vi "new square 1.vi"(11 "Error In":errorcluster) -> ()   [LabVIEW 2019]
uses:
  <vilib>/Platform/TimedLoop/XDataNode/timing_clust.ctl
  <vilib>/Platform/TimedLoop/XDataNode/nitl_modes.ctl
  <vilib>/Platform/TimedLoop/XDataNode/wakeup.ctl
  Global.vi
  <vilib>/platform/TimedLoop/XDataNode/XDataNode.xnode
  <vilib>/Platform/TimedLoop/XDataNode/XDNodeRunTimeDep.lvlib
panel:
  out "x >= y?":bool
  in  "msec Delay":u32=500
  out "msec Low":dbl=400.0
  out "msec High":dbl=600.0
  out "Duty Cycle":dbl
  out "Frequency":dbl
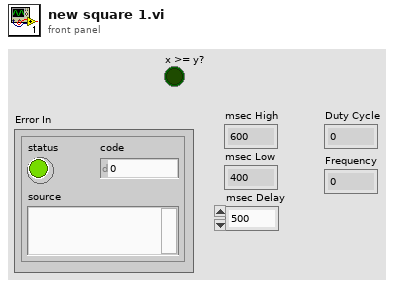
[diagram p1: front panel]
types:
  T1 = typedef "XDNodeRunTimeDep.lvlib/timing_clust.ctl" = cluster{"Expected End [f-1]":u64, "Actual End [f-1]":u64, "Finished Late? [f-1]":bool, "Expected End [i-1]":u64, "Actual End [i-1]":u64, "Finished Late? [i-1]":bool, "Expected Start [i]":u64, "Actual Start [i]":u64, "Expected Start [f]":u64, "Actual Start [f]":u64, "Source Name":string, "Structure Name":string, "Period":i64, "Deadline":i64, "Offset":i64, "Start":i64, "Priority":i32, "Timeout":i32, "Mode":T2, "Wakeup Reason":T3, "Error":errorcluster, "Source Type":string, "Secondary Source Type":string, "Global End Time":u64, "Global Start Time":u64, "Frame Duration":u64, "Iteration Duration":u64, "Assigned CPU":i32, "I/O Scan Engine Mode":u32}
  T2 = typedef "XDNodeRunTimeDep.lvlib/nitl_modes.ctl" = enum32{"No Change", "Process missed periods, maintain original phase", "Discard missed periods, maintain original phase", "Process missed periods, ignore original phase", "Discard missed periods, ignore original phase"}
  T3 = typedef "XDNodeRunTimeDep.lvlib/wakeup.ctl" = enum32{"Normal", "Aborted", "Asynchronous wakeup", "Timing source error", "Timed loop error", "Timeout"}
  T4 = cluster{"Frequency (Hz)":dbl, "Delay":dbl, "Duty cycle %":dbl}
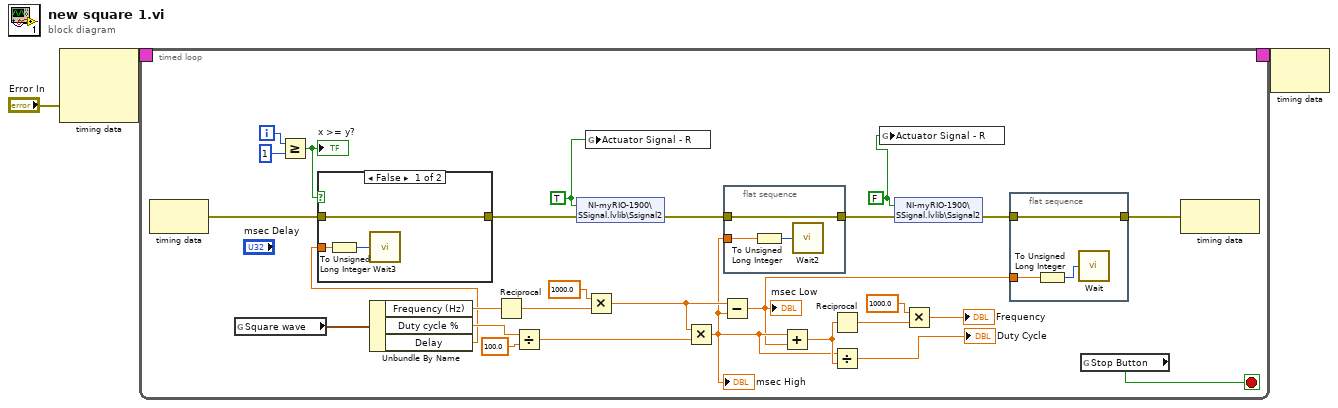
[diagram p0: block diagram]
diagram:
  n1 = node-c288("Error In") -> (w3:T1)  [unwired: 2 in]
  n2 = timed-loop {
    timing: w3 -> [_]
    timing-out: [_] -> w2
    i -> [w23]
    stop <- w25 stop-if-true
    w5 = FALSE ("DO0")
    w4 = TRUE ("DO0")
    n3 = node-c288() -> (w20:errorcluster)  [unwired: 1 in]
    n4 = global read "Global.vi" "Square wave"() -> (w18:T4)
    n5 = Greater Or Equal?(x=w23, y=1 ("x")) -> (x >= y?=w22:bool)
    "x >= y?" <- w22
    n6 = Unbundle By Name(w18) -> ("Frequency (Hz)"=w17:dbl, "Duty cycle %"=w15:dbl, "Delay"=w6:dbl)
    n7 = case shown="False" w22 {
      tunnel: w6 -> [w39 _]
      tunnel: w20 -> [w38 w40]
      tunnel: [w38 w40] -> w21
      frame False {
        n8 = To Unsigned Long Integer(number=w39) -> (unsigned 32bit integer=w37:u32)
        n9 = call "Wait3"("Count(mSec)"=w37) -> ()  [unwired: 1 out]
      }
      frame True {
      }
    }
    n10 = Reciprocal(x=w17) -> (1/x=w16:dbl)
    n11 = Divide(x=w15, y=100.0) -> (x/y=w13:dbl)
    n12 = shared-variable "NI-myRIO-1900\\SSignal.lvlib\\Ssignal2"(w4, error in=w21) -> (error out=w29:errorcluster)
    n13 = global write "Global.vi" "Actuator Signal - R"(w4) -> ()
    n14 = Multiply(x=1000.0, y=w16) -> (x*y=w14:dbl)
    n15 = Multiply(x=w14, y=w13) -> (x*y=w10:dbl)
    "msec High" <- w10
    n16 = Subtract(x=w14, y=w10) -> (x-y=w9:dbl)
    "msec Low" <- w9
    n17 = flat-sequence {
      tunnel: w10 -> [w43]
      tunnel: w29 -> [w42]
      tunnel: [w42] -> w28
      frame #0 {
        n18 = To Unsigned Long Integer(number=w43) -> (unsigned 32bit integer=w41:u32)
        n19 = call "Wait2"("Count(mSec)"=w41) -> ()  [unwired: 1 out]
      }
    }
    n20 = Add(x=w10, y=w9) -> (x+y=w26:dbl)
    n21 = Reciprocal(x=w26) -> (1/x=w30:dbl)
    n22 = Divide(x=w10, y=w26) -> (x/y=→"Duty Cycle":dbl)
    n23 = global write "Global.vi" "Actuator Signal - R"(w5) -> ()
    n24 = shared-variable "NI-myRIO-1900\\SSignal.lvlib\\Ssignal2"(w5, error in=w28) -> (error out=w27:errorcluster)
    n25 = Multiply(x=1000.0, y=w30) -> (x*y=→"Frequency":dbl)
    n26 = flat-sequence {
      tunnel: w27 -> [w46]
      tunnel: [w46] -> w19
      tunnel: w9 -> [w45]
      frame #0 {
        n27 = To Unsigned Long Integer(number=w45) -> (unsigned 32bit integer=w44:u32)
        n28 = call "Wait"("Count(mSec)"=w44) -> ()  [unwired: 1 out]
      }
    }
    n29 = global read "Global.vi" "Stop Button"() -> (w25:bool)
    n30 = node-c288(w19) -> ()  [unwired: 1 out]
  }
  n31 = node-c288(w2) -> ()  [unwired: 1 out]
